vi "CFG Convert Variant to String.vi"(0 "Key Cluster":T1, 5 "Value (Variant)":variant, 11 "error In":errorcluster) -> (4 "Value (Str)":string, 15 "error out":errorcluster)   [LabVIEW 2012]
uses:
  Type Defs/CFG Key Cluster.ctl
  Type Defs/CFG Tag Type Enum.ctl
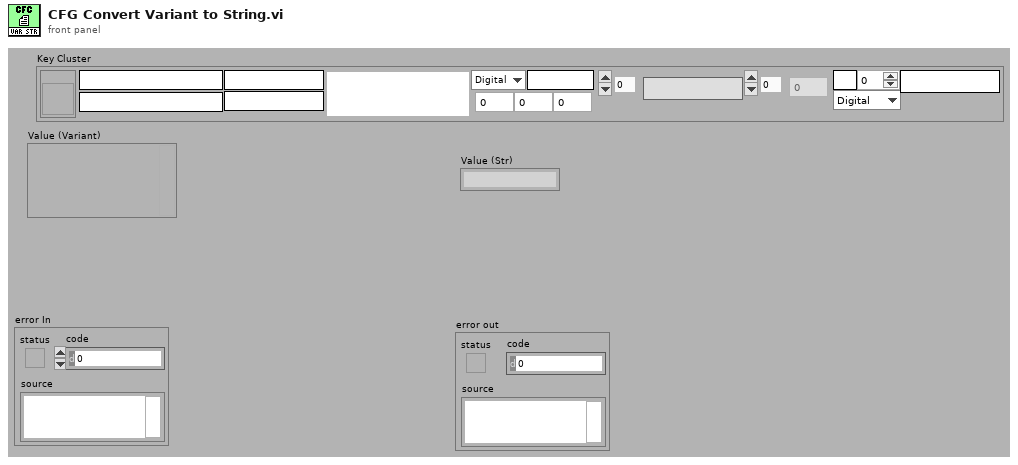
[diagram p1: front panel]
types:
  T1 = typedef "CFG Key Cluster.ctl" = cluster{"Strings []":string[], "Disabled Items []":i32[], "Value":variant, "Format String":string, "Tag":string, "Type":T2, "Section":string, " Ctl Ref":refnum<vi>, "Data Range":cluster{"Minimum":dbl, "Maximum":dbl, "Increment":dbl}, "Unit":string, "Special Instructions":string, "Delimiter(s)":string, "Dimensions":i32, "Element Type":T2, "Array Value String":string}
  T2 = typedef "CFG Tag Type Enum.ctl" = enum16{"Digital", "Slide", "Enum", "Boolean", "String", "Path", "Array", "VISAResourceName", "DAQmxName", "Cluster"}
  T3 = typedef "CFG DAQmx Type Enum.ctl" = enum16{"Analog Input", "Analog Output", "Digital Input", "Digital Output", "Counter Input", "Counter Output", "Terminal", ""}
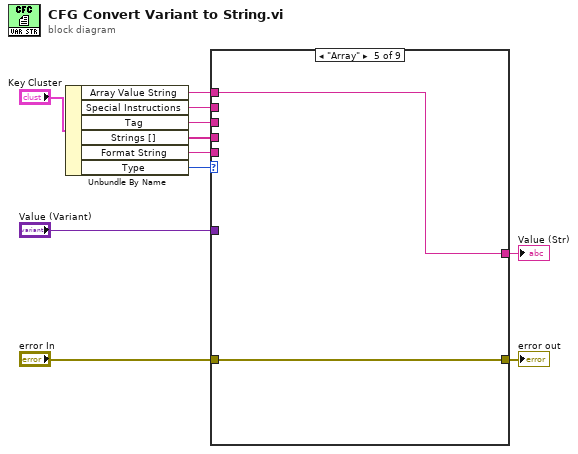
[diagram p0: block diagram]
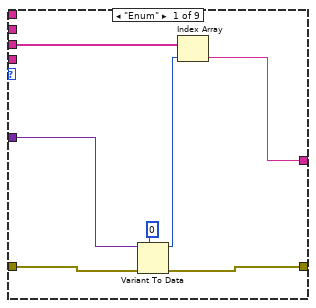
[diagram p2: hidden frame]
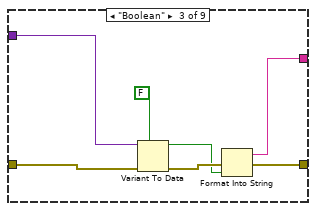
[diagram p4: hidden frame]
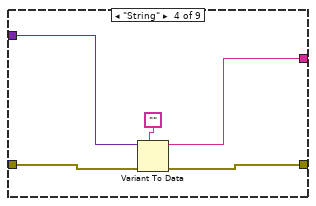
[diagram p5: hidden frame]
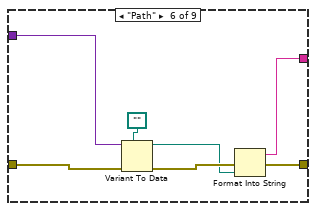
[diagram p6: hidden frame]
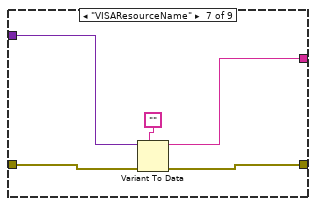
[diagram p7: hidden frame]
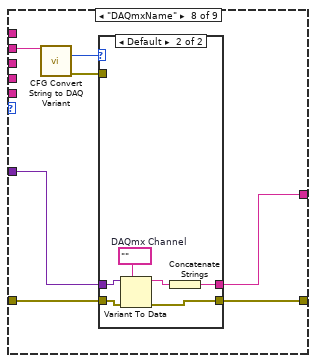
[diagram p8: hidden frame]
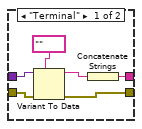
[diagram p9: hidden frame]
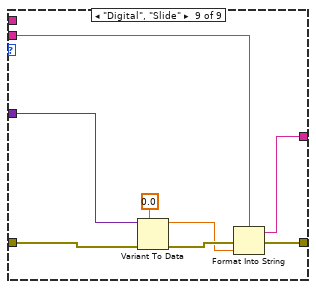
[diagram p10: hidden frame]
diagram:
  n1 = Unbundle By Name("Key Cluster") -> ("Array Value String"=w1:string, "Special Instructions"=w2:string, "Tag"=w3:string, "Strings []"=w4:string[], "Format String"=w5:string, "Type"=w7:T2)
  n2 = case shown="\"Array\"" w7 {
    tunnel: "Value (Variant)" -> [w15 _ w25 w30 _ w39 w44 w48 w71]
    tunnel: "error In" -> [w16 w19 w26 w31 w32 w40 w45 w52 w72]
    tunnel: [w12 w19 w22 w27 w32 w36 w42 w51 w68] -> w9
    tunnel: [w13 _ w20 w28 w33 w34 w41 w47 w65] -> w6
    tunnel: w5 -> [_ _ _ _ _ _ _ _ w66]
    tunnel: w4 -> [w14 _ _ _ _ _ _ _ _]
    tunnel: w3 -> [_ _ _ _ _ _ _ _ _]
    tunnel: w2 -> [_ _ _ _ _ _ _ w50 _]
    tunnel: w1 -> [_ _ _ _ w33 _ _ _ _]
    frame "Enum" {
      n3 = Variant To Data(error in=w16, type=0, Variant=w15) -> (data=w18:i32, error out=w12:errorcluster)
      n4 = Index Array(array=w14, index=w18) -> (element=w13:string)
    }
    frame "Cluster" {
    }
    frame "Boolean" {
      n5 = Variant To Data(error in=w26, type=FALSE ("default value"), Variant=w25) -> (data=w21:bool, error out=w23:errorcluster)
      n6 = Format Into String(error in=w23, w21) -> (resulting string=w20:string, error out=w22:errorcluster)  [unwired: 2 in]
    }
    frame "String" {
      n7 = Variant To Data(error in=w31, type="", Variant=w30) -> (data=w28:string, error out=w27:errorcluster)
    }
    frame "Array" {
    }
    frame "Path" {
      n8 = Variant To Data(error in=w40, type=path "", Variant=w39) -> (data=w35:path, error out=w37:errorcluster)
      n9 = Format Into String(error in=w37, w35) -> (resulting string=w34:string, error out=w36:errorcluster)  [unwired: 2 in]
    }
    frame "VISAResourceName" {
      n10 = Variant To Data(error in=w45, type="", Variant=w44) -> (data=w41:string, error out=w42:errorcluster)
    }
    frame "DAQmxName" {
      n11 = call "CFG Convert String to DAQ Variant.vi"("Special Instructions"=w50) -> ("DAQmx Type"=w49:T3, "error out"=w46:errorcluster)  [unwired: 3 in, 10 out]
      n12 = case shown="Default" w49 {
        tunnel: w52 -> [w58 w61]
        tunnel: [w55 w59] -> w47
        tunnel: [w57 w60] -> w51
        tunnel: w48 -> [w54 w62]
        tunnel: w46 -> [_ _]
        frame "Terminal" {
          n13 = Variant To Data(error in=w58, type=tag "" ("Terminal"), Variant=w54) -> (data=w56:tag, error out=w57:errorcluster)
          n14 = Concatenate Strings(w56) -> (w55:string)
        }
        frame Default {
          w63 = tag ""  # DAQmx Channel
          n15 = Variant To Data(error in=w61, type=w63, Variant=w62) -> (data=w64:tag, error out=w60:errorcluster)
          n16 = Concatenate Strings(w64) -> (w59:string)
        }
      }
    }
    frame "Digital", "Slide" {
      n17 = Variant To Data(error in=w72, type=0.0, Variant=w71) -> (data=w67:dbl, error out=w69:errorcluster)
      n18 = Format Into String(format string=w66, error in=w69, w67) -> (resulting string=w65:string, error out=w68:errorcluster)  [unwired: 1 in]
    }
  }
  "error out" <- w9
  "Value (Str)" <- w6
